vi "YPR char to data.vi"(8 "Error In":errorcluster, 10 "YPR char value":u8[](array[numeric])) -> (0 "Error Out":errorcluster, 2 "YPR data":cluster{"Yaw":sgl, "Pitch":sgl, "Roll":sgl})   [LabVIEW 2016]
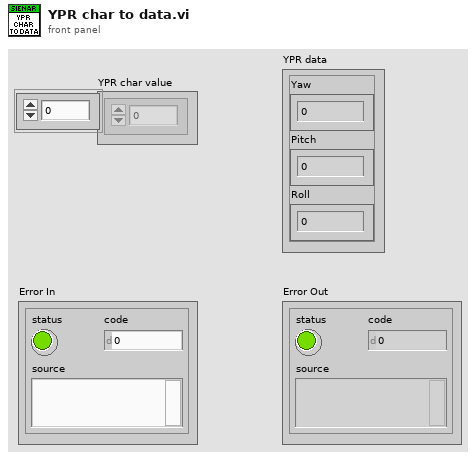
[diagram p1: front panel]
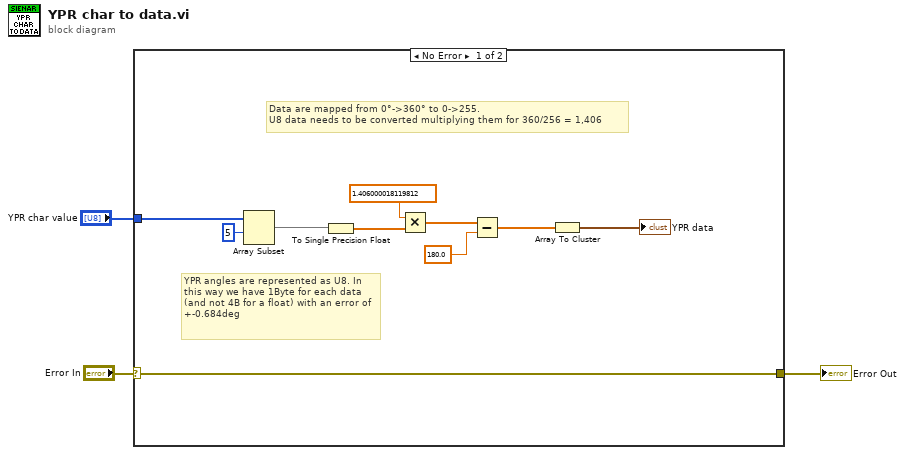
[diagram p0: block diagram]
diagram:
  n1 = case shown="No Error" "Error In" {
    selector: "Error In" -> [w12 w14]
    tunnel: [w12 w14] -> w2
    tunnel: "YPR char value" -> [w11 _]
    frame No Error {
      # "Data are mapped from 0°->360° to 0->255.\nU8 data needs to be converted multiplying them for 360/256 = 1,406"
      # "YPR angles are represented as U8. In this way we have 1Byte for each data (and not 4B for a float) with an error of +-0.684deg"
      n2 = Array Subset(array=w11, index=5) -> (w10:u8[])  [unwired: 1 in]
      n3 = To Single Precision Float(number=w10) -> (single precision float=w9:sgl[])
      n4 = Multiply(x=sgl 1.406, y=w9) -> (x*y=w5:sgl[])
      n5 = Subtract(x=w5, y=sgl 180.0) -> (x-y=w4:sgl[])
      n6 = Array To Cluster(array=w4) -> (cluster=→"YPR data":cluster{"[0]":sgl, "[1]":sgl, "[2]":sgl})
    }
    frame Error {
    }
  }
  "Error Out" <- w2
